vi "Save for Previous Version.vi"(8 "error in (no error)":errorcluster, 10 "LabVIEW Version":string, 11 "LabVIEW Project File in":refnum<class "LabVIEW Project File.lvclass">) -> (0 "error out":errorcluster, 1 "Errors":string, 2 "Warnings":string, 3 "LabVIEW Project File out":refnum<class "LabVIEW Project File.lvclass">)   [LabVIEW 2020, in "Save for Previous Version.lvlib" / "LabVIEW Project File.lvclass"]
uses:
  LabVIEW Project File.lvclass
  \\Mac\Home/JKI/GitHub/vipm-io/a-version-explorer-for-labview/experiments/save-for-previous-version/source/File/File.lvclass/File.lvclass
  File/File.lvclass/File.lvclass/File.ctl
  File/File.lvclass/Read Path.vi
  LabVIEW File/LabVIEW File.lvclass
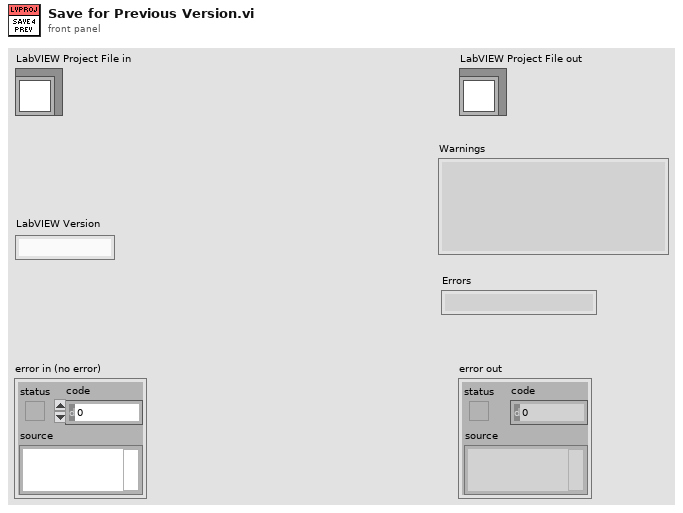
[diagram p1: front panel]
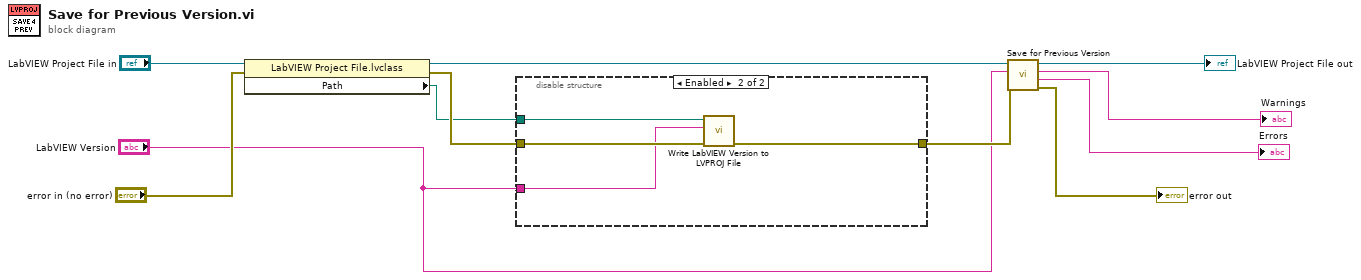
[diagram p0: block diagram]
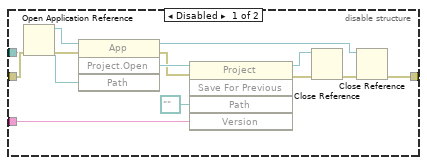
[diagram p2: hidden frame]
diagram:
  n1 = property class="LabVIEW Project File.lvclass"(reference="LabVIEW Project File in", error in="error in (no error)") -> (reference out=w11:refnum<class "LabVIEW Project File.lvclass">, error out=w7:errorcluster, "Path"=w1:path)
  n2 = disable-structure shown="Enabled" {
    disable-tunnel: w7 -> [w16 w28]
    disable-tunnel: [w15 w25] -> w6
    disable-tunnel: "LabVIEW Version" -> [w14 w27]
    disable-tunnel: w1 -> [w12 w26]
    frame Disabled {
      n3 = Open Application Reference(8:w16) -> (0:w24:errorcluster, 3:w23:refnum<vi>)  [unwired: 3 in]
      n4 = invoke class="App" method="Project.Open"(reference=w23, error in=w24, "Path"=w12) -> (reference out=w17:refnum<vi>, error out=w21:errorcluster, "Project:Open"=w22:refnum<vi>)  [unwired: 1 in, 1 out]
      n5 = invoke class="Project" method="Save For Previous"(reference=w22, error in=w21, "Path"=path "", "Version"=w14) -> (reference out=w19:refnum<vi>, error out=w20:errorcluster)  [unwired: 1 in, 3 out]
      n6 = Close Reference(reference=w19, error in (no error)=w20) -> (error out=w18:errorcluster)
      n7 = Close Reference(reference=w17, error in (no error)=w18) -> (error out=w15:errorcluster)
    }
    frame Enabled {
      n8 = call "Write LabVIEW Version to LVPROJ File.vi"("error in"=w28, "LabVIEW Version"=w27, "Project File Path"=w26) -> ("error out"=w25:errorcluster)  [unwired: 7 in, 1 out]
    }
  }
  n9 = call-parent "Save for Previous Version.vi"("error in (no error)"=w6, "LabVIEW Version"="LabVIEW Version", "LabVIEW File in"=w11) -> ("error out"=→"error out":errorcluster, "Errors"=→"Errors":string, "Warnings"=→"Warnings":string, "LabVIEW File out"=→"LabVIEW Project File out":refnum<class "LabVIEW Project File.lvclass">)  [unwired: 5 in]
